vi "DSF.UDP.Transfer.Create.vi"(5 "Port":u16, 7 "IP Address":string="localhost", 8 "error in (no error)":errorcluster, 9 "Direction":T5, 10 "Name":string, 11 "Channel Descriptors":T1[](array[typedef]) {"VS Channel Ref" format="%016x"; "Channel Parameters"."offset" format="%d bytes"}) -> (0 "error out":errorcluster, 3 "UDP Transfer out":refnum<class "DSF.UDP.Configuration.Transfer.lvclass">)   [LabVIEW 2016, in "DSF.UDP.Configuration.Transfer.lvclass"]
uses:
  DSF.UDP.Configuration.Transfer.lvclass
  C:/Git/SourceTree/DSF/Source/Shared/Classes/Transfer/DSF.Shared.Configuration.Transfer.lvclass
  Source/Shared/Typedefs/DSF.Shared.Typedefs.Direction.ctl
  Source/Shared/Typedefs/DSF.Shared.Typedefs.Configuration.Transfer.Channel Descriptor.ctl
  Source/Shared/Typedefs/DSF.Shared.Typedefs.Configuration.Transfer.Channel Parameters.ctl
  Source/Shared/Typedefs/DSF.Shared.Typedefs.Data Type.ctl
  <vilib>/NI Veristand/Custom Device API/Custom Device Item Ref.ctl
  DSF.UDP.Configuration.Transfer.lvclass/DSF.UDP.Configuration.Transfer.ctl
  Source/Shared/Classes/Transfer/DSF.Shared.Configuration.Transfer.lvclass
  Source/DSF.Shared.lvlib
  <vilib>/NI Veristand/Custom Device API/Custom Device API.lvlib
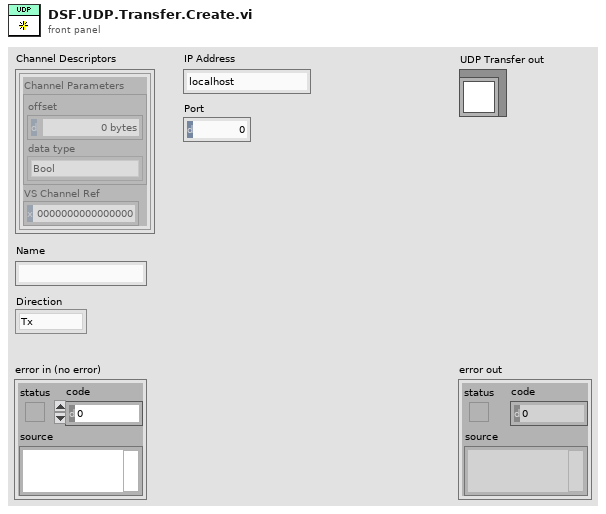
[diagram p1: front panel]
types:
  T1 = typedef "DSF.Shared.lvlib/DSF.Shared.Typedefs.Configuration.Transfer.Channel Descriptor.ctl" = cluster{"Channel Parameters":T2, "VS Channel Ref":T4}
  T2 = typedef "DSF.Shared.lvlib/DSF.Shared.Typedefs.Configuration.Transfer.Channel Parameters.ctl" = cluster{"offset":u64, "data type":T3}
  T3 = typedef "DSF.Shared.lvlib/DSF.Shared.Typedefs.Data Type.ctl" = enum8{"Bool", "SGL", "DBL", "I8", "I16", "I32", "I64", "U8", "U16", "U32", "U64"}
  T4 = typedef "Custom Device API.lvlib/Custom Device Item Ref.ctl" = u64
  T5 = typedef "DSF.Shared.lvlib/DSF.Shared.Typedefs.Direction.ctl" = enum16{"Tx", "Rx"}
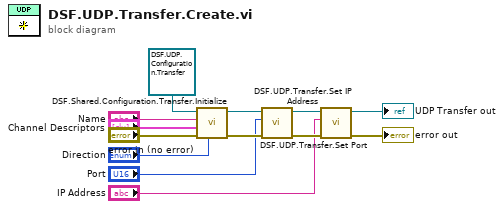
[diagram p0: block diagram]
diagram:
  n1 = call "DSF.Shared.Configuration.Transfer.Initialize.vi"("Direction"="Direction", "error in (no error)"="error in (no error)", "Channel Descriptors"="Channel Descriptors", "Name"="Name", "Transfer Configuration in"=refnum<class "DSF.UDP.Configuration.Transfer.lvclass"> refnum ("UDP Transfer in")) -> ("error out"=w8:errorcluster, "Transfer Configuration out"=w7:refnum<class "DSF.UDP.Configuration.Transfer.lvclass">)  [unwired: 5 in]
  n2 = call "DSF.UDP.Transfer.Set Port.vi"("error in (no error)"=w8, "Port"="Port", "UDP Transfer in"=w7) -> ("error out"=w5:errorcluster, "UDP Transfer out"=w6:refnum<class "DSF.UDP.Configuration.Transfer.lvclass">)  [unwired: 7 in]
  n3 = call "DSF.UDP.Transfer.Set IP Address.vi"("error in (no error)"=w5, "IP Address"="IP Address", "UDP Transfer in"=w6) -> ("error out"=→"error out":errorcluster, "UDP Transfer out"=→"UDP Transfer out":refnum<class "DSF.UDP.Configuration.Transfer.lvclass">)  [unwired: 7 in]
